vi "wsCheckIfRegMsgOK.vi"(8 "error in (no error)":errorcluster, 10 "msgCounter":string, 11 "References":T1) -> (0 "error out":errorcluster, 2 "raw result":string, 3 "Success?":bool)   [LabVIEW 2018, in "HASS-LV-WS_integration.lvlib"]
uses:
  HASS-LV-WS_integration.lvlib
  TypeDef/ReferencesTypeDef.ctl
  TypeDef/QueueTypeDef.ctl
  TypeDef/EventTypeDef.ctl
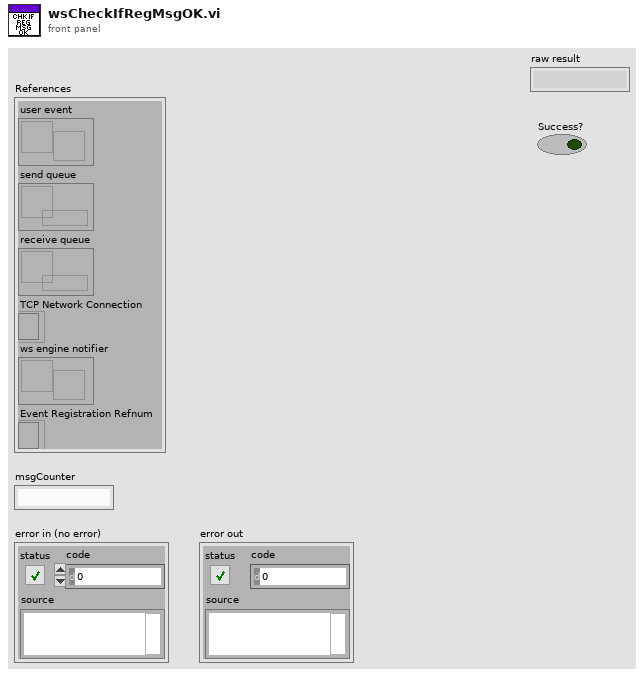
[diagram p1: front panel]
types:
  T1 = typedef "HASS-LV-WS_integration.lvlib/ReferencesTypeDef.ctl" = cluster{"user event":refnum<user-event>, "send queue":refnum<queue>, "receive queue":refnum<queue>, "TCP Network Connection":refnum<k5>, "ws engine notifier ":refnum<notifier>, "Event Registration Refnum":refnum<event-registration>}
  T2 = typedef "HASS-LV-WS_integration.lvlib/EventTypeDef.ctl" = cluster{"Data":variant, "Command":string}
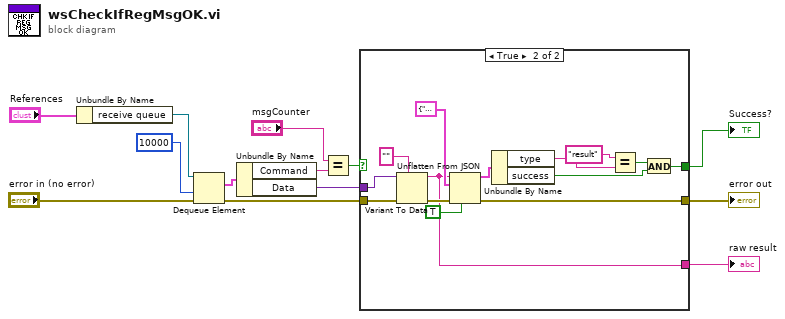
[diagram p0: block diagram]
diagram:
  n1 = Unbundle By Name("References") -> ("receive queue"=w12:refnum<queue>)
  n2 = Dequeue Element(queue=w12, timeout in ms (-1)=10000, error in (no error)="error in (no error)") -> (element=w4:T2, error out=w10:errorcluster)  [unwired: 2 out]
  n3 = Unbundle By Name(w4) -> ("Command"=w5:string, "Data"=w7:variant)
  n4 = Equal?(x="msgCounter", y=w5) -> (x = y?=w8:bool)
  n5 = case shown="True" w8 {
    tunnel: w7 -> [_ w28]
    tunnel: [_ w20] -> w9
    tunnel: w10 -> [w14 w19]
    tunnel: [w14 w18] -> w11
    tunnel: [_ w15] -> w1
    frame False {
    }
    frame True {
      n6 = Variant To Data(error in=w19, type="", Variant=w28) -> (data=w15:string, error out=w26:errorcluster)
      n7 = Unflatten From JSON(JSON string=w15, type and defaults=cluster{"type":string, "success":bool, "id":i32} {"type"="", "success"=FALSE, "id"=0}, default null elements? (F)=TRUE, error in (no error)=w26) -> (value=w24:cluster{"type":string, "success":bool, "id":i32}, error out=w18:errorcluster)  [unwired: 3 in]
      n8 = Unbundle By Name(w24) -> ("type"=w23:string, "success"=w17:bool)
      n9 = Equal?(x="result", y=w23) -> (x = y?=w21:bool)
      n10 = And(x=w21, y=w17) -> (x .and. y?=w20:bool)
    }
  }
  "error out" <- w11
  "Success?" <- w9
  "raw result" <- w1
